vi "File Write Binary File.vi"(4 "Input Varaint":variant, 6 "字节顺序":T1(ring)=enum."little-endian", 7 "prepend array or string size? (T)":bool, 8 "error in":errorcluster, 9 "access (0:read/write)":enum16{"read/write", "read-only", "write-only"}(ring)=enum."write-only", 10 "operation (0:open)":T2(ring)=enum."create", 11 "File path":path) -> (0 "error out":errorcluster, 1 "cancelled":bool, 3 "path":path)   [LabVIEW 2018]
doc: "将数据数组写入字节流二进制文件。默认情况下，VI被配置为写入8字节Little Endian数据（双精度长整型DBL）。如要修改采样数据写入文件的方式，修改字节顺序，并使用编程>>数值>>转换选板上的VI将数据数组(DBL)的表示法改为I8（单字节）、I16（双字节）或I32（4字节）。用“读取二进制文件”VI读取文件。"
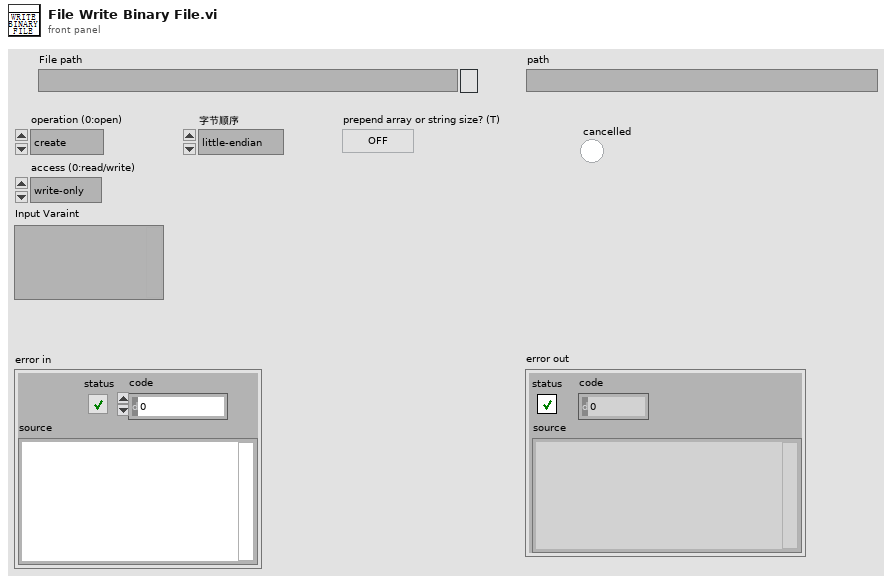
[diagram p1: front panel]
types:
  T1 = enum16{"big-endian, network order", "native, host order", "little-endian"}
  T2 = enum16{"open", "replace", "create", "open or create", "replace or create", "replace or create with confirmation"}
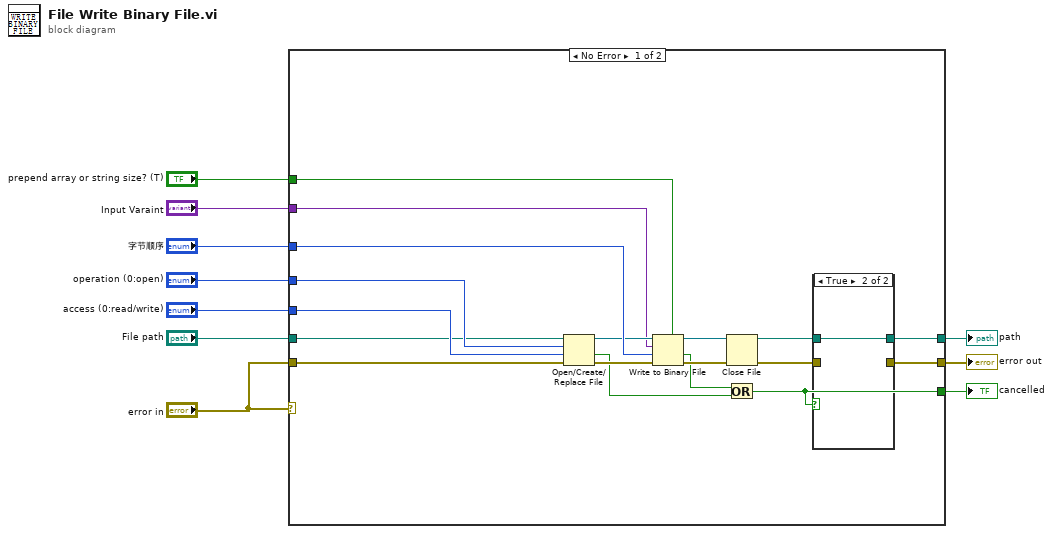
[diagram p0: block diagram]
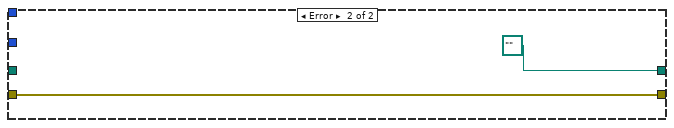
[diagram p3: hidden frame]
diagram:
  n1 = case shown="No Error" "error in" {
    tunnel: [w13 path "" ("path")] -> w10
    tunnel: "error in" -> [w28 w32]
    tunnel: [w12 w32] -> w9
    tunnel: "access (0:read/write)" -> [w27 _]
    tunnel: "operation (0:open)" -> [w26 _]
    tunnel: "File path" -> [w25 _]
    tunnel: "prepend array or string size? (T)" -> [w24 _]
    tunnel: "字节顺序" -> [w23 _]
    tunnel: [w15 _] -> w2
    tunnel: "Input Varaint" -> [w18 _]
    frame No Error {
      n2 = Open/Create/Replace File(file path (use dialog)=w25, error in=w28, operation (0:open)=w26, access (0:read/write)=w27) -> (refnum out=w19:refnum<file>, cancelled=w16:bool, error out=w20:errorcluster)  [unwired: 2 in]
      n3 = Write to Binary File(file (use dialog)=w19, data=w18, error in=w20, 5:w24, 9:w23) -> (refnum out=w22:refnum<file>, cancelled=w17:bool, error out=w21:errorcluster)  [unwired: 1 in]
      n4 = Close File(refnum=w22, error in=w21) -> (path=w14:path, error out=w11:errorcluster)
      n5 = Or(x=w17, y=w16) -> (x .or. y?=w15:bool)
      n6 = case shown="True" w15 {
        tunnel: w14 -> [w29 w31]
        tunnel: [w29 w31] -> w13
        tunnel: [w30 _] -> w12
        tunnel: w11 -> [w30 _]
        frame False {
        }
        frame True {
        }
      }
    }
    frame Error {
    }
  }
  "path" <- w10
  "error out" <- w9
  "cancelled" <- w2
